vi "g_CipHolderConstants.vi"() -> ()   [LabVIEW 2014]
panel:
  in  "#Slots Y":dbl=3.0
  in  "#Slots X":dbl=5.0
  out "Home Y":dbl
  out "Home X":dbl
  in  "Length Chipslot":dbl=10.0
  in  "Width Chipslot":dbl=8.0
  in  "Length Y":dbl=66.0
  in  "Width X":dbl=40.0
  # "Dimensions in mm"
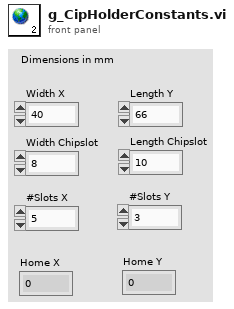
[diagram p1: front panel]
diagram:
